vi "Xml_Load_Excit_Table.vi"(7 "Version String":string, 8 "error in (no error)":errorcluster, 10 "XML Path":path=path "D:/TEST.xml", 11 "Refnum Clust":refnum<vi>) -> (0 "error out":errorcluster)   [LabVIEW 2017]
uses:
  controls/EXCIT_Table.ctl
panel:
  in  "EXCIT Table":T1={"Number of Excits"=0, "Number of Ejects"=0, "Sampling Frequency"=0.0, "Waveforms Table"=[["Excit1", "name", "Swift", "0.5", "1200", "70", "150", "550", "0", "0", "0"]]}
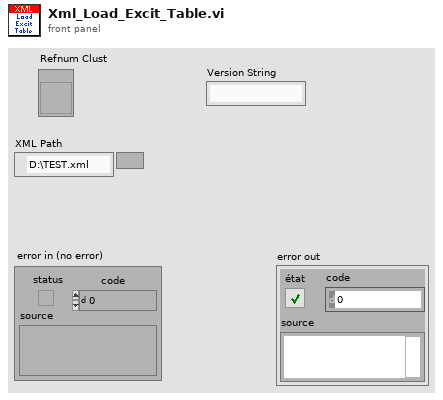
[diagram p1: front panel]
types:
  T1 = typedef "EXCIT_Table.ctl" = cluster{"Number of Excits":u16, "Number of Ejects":u16, "Sampling Frequency":dbl, "Waveforms Table":string[][]}
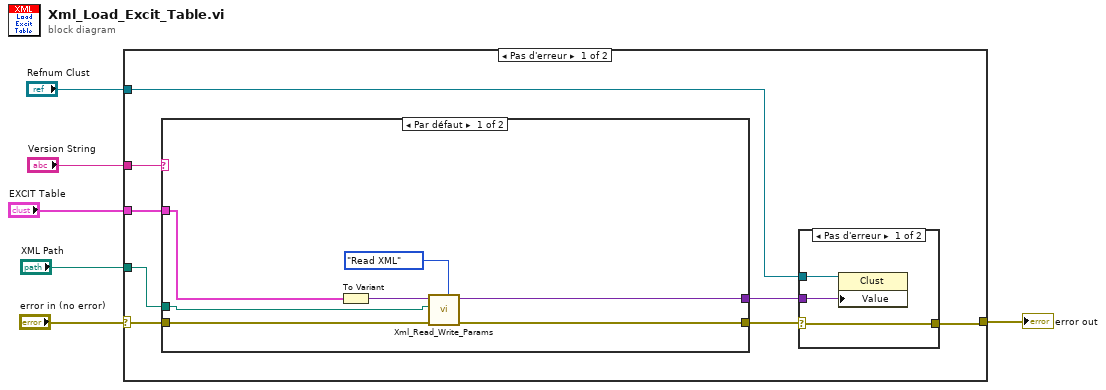
[diagram p0: block diagram]
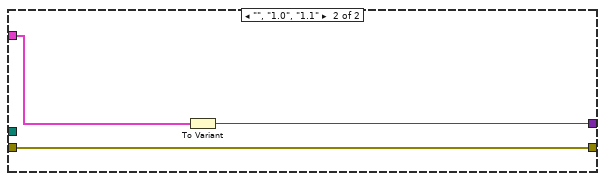
[diagram p3: hidden frame]
diagram:
  n1 = case shown="Pas d'erreur" "error in (no error)" {
    selector: "error in (no error)" -> [w14 w29]
    tunnel: [w9 w29] -> w6
    tunnel: "XML Path" -> [w13 _]
    tunnel: "Version String" -> [w12 _]
    tunnel: "Refnum Clust" -> [w7 _]
    tunnel: "EXCIT Table" -> [w11 _]
    frame No Error {
      n2 = case shown="Par défaut" w12 {
        tunnel: w14 -> [w23 w27]
        tunnel: [w21 w27] -> w10
        tunnel: [w22 w28] -> w8
        tunnel: w13 -> [w20 _]
        tunnel: w11 -> [w19 w26]
        frame Default {
          n3 = To Variant(anything=w19) -> (Variant=w24:variant)
          n4 = call "Xml_Read_Write_Params.vi"("Variant"=w24, "XML Path"=w20, "error in (no error)"=w23, "Command"=enum16{"Read XML", "Set", "Get", "Write XML"}."Read XML") -> ("Variant Output"=w22:variant, "error out"=w21:errorcluster)  [unwired: 3 in, 1 out]
        }
        frame "", "1.0", "1.1" {
          n5 = To Variant(anything=w26) -> (Variant=w28:variant)
        }
      }
      n6 = case shown="Pas d'erreur" w10 {
        selector: w10 -> [w16 w18]
        tunnel: w7 -> [w17 _]
        tunnel: [w16 w18] -> w9
        tunnel: w8 -> [w15 _]
        frame No Error {
          n7 = property class="Clust"(reference=w17, "Value"=w15) -> ()  [unwired: 1 in, 2 out]
        }
        frame Error {
        }
      }
    }
    frame Error {
    }
  }
  "error out" <- w6
